vi "GT Sdram To Flash.vi"(8 "error in (no error)":errorcluster caption="错误输入（无错误）", 10 "pRetry":i32, 11 "cardNum":i16) -> (0 "error out":errorcluster caption="错误输出", 2 "pRetry out":i32, 3 "function return":i16)   [LabVIEW 2020, in "gts1.lvlib"]
doc: "GT_API GT_SdramToFlash(short cardNum,long *pRetry=NULL);"
uses:
  gts1.lvlib
  dll/32bit/multi_card/gts.dll
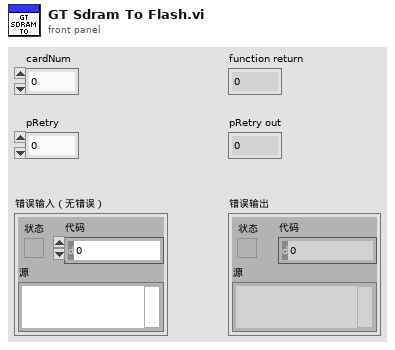
[diagram p1: front panel]
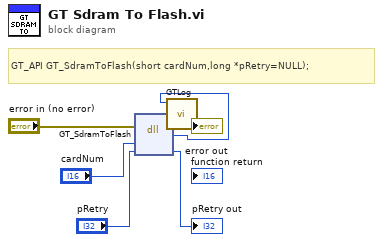
[diagram p0: block diagram]
diagram:
  # "GT_API GT_SdramToFlash(short cardNum,long *pRetry=NULL);"
  n1 = dll-call lib="C:/1228/dll/32bit/multi_card/gts.dll" fn="GT_SdramToFlash"(error in="error in (no error)", "cardNum"="cardNum", "pRetry"="pRetry") -> (error out=w3:errorcluster, w1:i16, "pRetry"=→"pRetry out":i32)  [unwired: 3 in, 1 out]
  n2 = call "GTLog.vi"("error in (no error)"=w3, "Numeric"=w1) -> ("error out"=→"error out":errorcluster)  [unwired: 9 in]
